vi "运维调试_采配水V4-华南所.vi"() -> ()   [LabVIEW 2016, in "PLC.lvlib"]
uses:
  PLC.lvlib
  control/switch.ctl
  <vilib>/Plasmionique/MB Master/MB_Master/MB_Master.lvclass
  <vilib>/Utility/miscctls.llb/LVPointTypeDef.ctl
  <vilib>/Plasmionique/MB Master/MB_Master_Serial/MB_Master_Serial.lvclass
  C:/Program Files (x86)/National Instruments/LabVIEW 2016/vi.lib/Plasmionique/MB Master/MB_Master/MB_Master.lvclass
  <vilib>/Plasmionique/MB Master/MB_Master_TCP/MB_Master_TCP.lvclass
  <vilib>/Instr/_visa.llb/VISA Configure Serial Port (Instr).vi
  <vilib>/Plasmionique/MB Master/MB Master.lvlib
panel:
  out "R138":i16 caption="水槽搅拌时间"
  out "R137":i16 caption="水槽润洗时间"
  out "X13":bool caption="三通道水槽3液位"
  out "X12":bool caption="三通道水槽2液位"
  out "X11":bool caption="三通道水槽1液位"
  in  "Y28":T1
  out "R41":i16
  in  "Y15":T1
  in  "Y16":T1
  in  "Y2":T1
  in  "Y3":T1
  in  "Y4":T1
  in  "Y5":T1
  in  "Y6":T1
  in  "Y7":T1
  in  "Y8":T1
  in  "Y9":T1
  in  "Y10":T1
  in  "Y11":T1
  in  "Y12":T1
  in  "Y0":T1
  in  "Y1":T1
  in  "Y13":T1
  in  "Y14":T1
  in  "Y17":T1
  in  "Y18":T1
  out "R13":u16
  out "R14":u16
  out "R15":u16
  out "R16":u16
  out "R17":u16
  out "R18":u16
  out "R19":u16
  out "R20":u16
  out "R21":u16
  out "R22":u16
  out "R23":u16
  out "R24":u16
  out "R25":u16
  out "R26":u16
  out "R27":u16
  out "R28":u16
  out "R29":u16
  out "R30":u16
  out "R31":u16
  in  "Y29":T1
  out "R42":i16
  in  "Y30":T1
  out "R43":u16
  in  "Y31":T1
  out "R44":u16
  in  "Y21":T1
  out "R34":u16
  in  "连接设置":bool
  in  "R136":u16(ring) caption="河水反冲洗模式" items=["泵保持", "泵交替"]
  out "R135":i16 caption="除藻时间"
  in  "R134":u16(ring) caption="除藻工作模式" items=["手动", "自动"]
  in  "R110":u16(ring) caption="反冲洗水体" items=["自来水", "河水"]
  in  "63μm反冲洗阀":bool
  out "供水压力":dbl format="%.4f"
  out "R111":i16 caption="三级水样池润洗时间"
  in  "三级过滤系统":bool
  out "R104":i16 caption="三级润洗时间"
  out "R103":i16 caption="二级润洗时间"
  out "R107":i16 caption="进气时间"
  out "Registers":u16[](array[numeric])
  out "R124":i16 caption="加标回收配水时间"
  in  "更新程序":T1
  out "R122":i16 caption="二级自来水清洗时间"
  out "R121":i16 caption="一级自来水清洗时间"
  out "R120":i16 caption="过滤自来水清洗时间"
  out "清洗次数":u16
  out "当前启动泵号":u16(ring) items=["1号泵", "2号泵"]
  out "R116":i16 caption="储水时间"
  in  "R113":u16(ring) caption="水箱储水水体" items=["自来水", "河水"]
  out "R112":i16 caption="二级水样池进样超时"
  out "配水压力":dbl format="%.4f"
  out "X2":bool caption="X1"
  out "采配水版本号":string
  out "R117":i16 caption="清洗频次设定"
  out "通讯故障":bool
  in  "R100":u16(ring) caption="采水泵工作模式" items=["泵1单泵单管路", "泵2单泵单管路", "潜水泵双泵双管路", "自吸泵双泵双管路"]
  out "X10":bool caption="氨氮水样池液位开关SL3"
  out "X9":bool caption="泵2过载报警_KM2"
  out "X8":bool caption="泵1过载报警_KM1"
  out "X7":bool caption="断电检测_PA"
  out "X6":bool caption="门禁开关_AS"
  out "X5":bool caption="烟雾检测_SA"
  out "X4":bool caption="浸水检测_WIA"
  out "X3":bool caption="水流开关_FS"
  out "X1":bool
  out "X0":bool caption="采样池液位开关_SL1"
  out "R109":i16 caption="外部反冲洗时间"
  out "R108":i16 caption="进样超时时间"
  out "R106":i16 caption="排液时间"
  out "R105":i16 caption="常规模式配水时间"
  out "R102":i16 caption="沉淀时间"
  out "R101":i16 caption="一级润洗时间"
  out "R2":i16
  out "R1":i16
  out "多列列表框":i32(listbox)
  in  "返回":T1
  in  "参数设置":T1
  in  "单步启动":T1
  in  "启动":T1
  in  "停止":T1
  out "集成报警信息":string
  # "s"
  # "流程计时："
  # "s"
  # "单步计时："
  # "MPa"
  # "配水压力："
  # "MPa"
  # "供水压力："
  # "S"
  # "S"
  # "S"
  # "S"
  # "S"
  # "S"
  # "S"
  # "S"
  # "S"
  # "S"
  # "S"
  # "S"
  # "S"
  # "次"
  # "S"
  # "S"
  # "S"
  # "S"
  # "S"
  # "S"
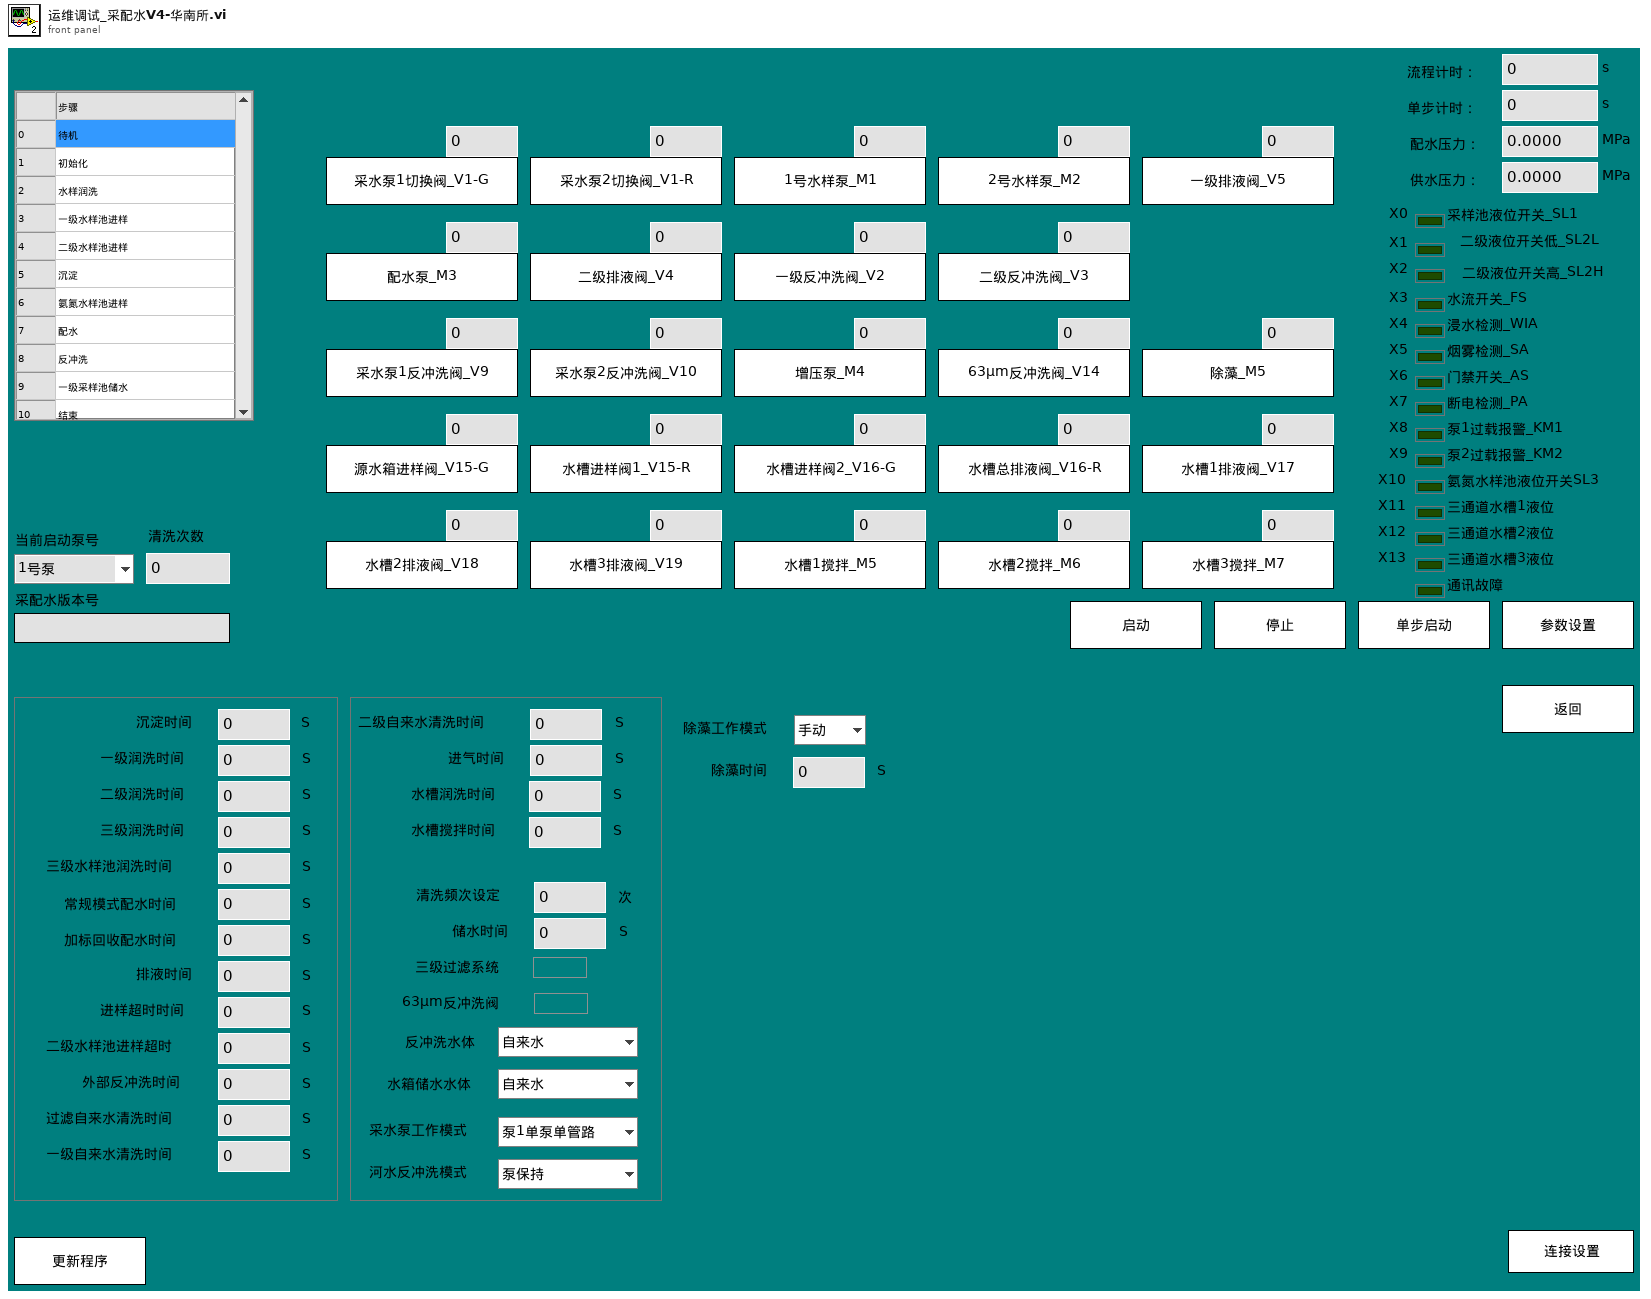
[diagram p1: front panel]
types:
  T1 = typedef "PLC.lvlib/switch.ctl" = bool
  T2 = typedef "参数.ctl" = cluster{"测试模式":enum16{"水样测试", "平行样测试", "集成干预测试", "加标回收"}, "参数启用":T3}
  T3 = typedef "启动参数.ctl" = cluster{"氨氮":bool, "总磷":bool, "总氮":bool, "多参数":bool, "CODmn":bool, "CODCr":bool, "氟化物":bool, "超标留样":bool, "重金属":bool, "挥发酚":bool}
  T4 = typedef "LVPointTypeDef.ctl" = cluster{"Horizontal":i16, "Vertical":i16}
  T5 = cluster{"命令":string, "数据":cluster{"starting address":u16, "holding register value":u16}}
  T6 = cluster{"R0":i16, "R1":i16, "R2":i16, "R3":i16, "R4":i16, "R5":i16, "R6":i16, "R7":i16, "R8":i16, "R9":i16, "R10":i16, "R11":i16, "R12":i16, "R13":i16, "R14":i16, "R15":i16, "R16":i16, "R17":i16, "R18":i16, "R19":i16, "R20":i16, "R21":i16, "R22":i16, "R23":i16, "R24":i16, "R25":i16, "R26":i16, "R27":i16, "R28":i16, "R29":i16, "R30":i16, "R31":i16, "R32":i16, "R33":i16, "R34":i16, "R35":i16, "R36":i16, "R37":i16, "R38":i16, "R39":i16, "R40":i16, "R41":i16, "R42":i16, "R43":i16, "R44":i16, "R45":i16, "R46":i16, "R47":i16, "R48":i16, "R49":i16, "R50":i16, "R51":i16, "R52":i16, "R53":i16, "R54":i16, "R55":i16, "R56":i16, "R57":i16, "R58":i16, "R59":i16, "R60":i16, "R61":i16, "R62":i16, "R63":i16, "R64":i16, "R65":i16, "R66":i16, "R67":i16, "R68":i16, "R69":i16, "R70":i16, "R71":i16, "R72":i16, "R73":i16, "R74":i16, "R75":i16, "R76":i16, "R77":i16, "R78":i16, "R79":i16}
  T7 = cluster{"seconds since 1Jan1904":timestamp, "table输入":string, string, "table输入":string}
  T8 = cluster{"命令":string, cluster{"starting address":u16, "holding register value":u16}}
  T9 = cluster{"命令":string, "数据":cluster{"starting address":u16, "holding register values":u16[]}}
  T10 = cluster{"命令":string, "data":cluster{"starting address":u16, "coil values":bool[]}}
  T11 = cluster{"测试模式":enum16{"水样测试", "平行样测试", "集成干预测试", "加标回收"}, "参数启用":T3}
  T12 = cluster{"baud rate (bps)":u32, "stop bits":u16, "parity":u16, "flow control":u16, "timeout":u32, "retries":i32}
  T13 = cluster{"starting address":u16, "holding register values":u16[]}
  T14 = cluster{"starting address":u16, "holding register value":u16}
  T15 = cluster{"starting address":u16, "coil values":bool[]}
  T16 = cluster{"连接类型":enum16{"串口", "TCP"}, "串口":string, "IP":string, "PORT":u16}
  T17 = cluster{"Registers[0]":u16, "Registers[1]":u16, "Registers[2]":u16, "Registers[3]":u16, "Registers[4]":u16, "Registers[5]":u16, "Registers[6]":u16, "Registers[7]":u16, "Registers[8]":u16, "Registers[9]":u16, "Registers[10]":u16, "Registers[11]":u16, "Registers[12]":u16, "Registers[13]":u16, "Registers[14]":u16, "Registers[15]":u16, "Registers[16]":u16, "Registers[17]":u16, "Registers[18]":u16, "Registers[19]":u16, "Registers[20]":u16, "Registers[21]":u16, "Registers[22]":u16, "Registers[23]":u16, "Registers[24]":u16, "Registers[25]":u16, "Registers[26]":u16, "Registers[27]":u16, "Registers[28]":u16, "Registers[29]":u16, "Registers[30]":u16, "Registers[31]":u16, "Registers[32]":u16, "Registers[33]":u16, "Registers[34]":u16, "Registers[35]":u16, "Registers[36]":u16, "Registers[37]":u16, "Registers[38]":u16, "Registers[39]":u16, "Registers[40]":u16, "Registers[41]":u16, "Registers[42]":u16, "Registers[43]":u16, "Registers[44]":u16, "Registers[45]":u16, "Registers[46]":u16, "Registers[47]":u16, "Registers[48]":u16, "Registers[49]":u16, "Registers[50]":u16, "Registers[51]":u16, "Registers[52]":u16, "Registers[53]":u16, "Registers[54]":u16, "Registers[55]":u16, "Registers[56]":u16, "Registers[57]":u16, "Registers[58]":u16, "Registers[59]":u16, "Registers[60]":u16, "Registers[61]":u16, "Registers[62]":u16, "Registers[63]":u16, "Registers[64]":u16, "Registers[65]":u16, "Registers[66]":u16, "Registers[67]":u16, "Registers[68]":u16, "Registers[69]":u16, "Registers[70]":u16, "Registers[71]":u16, "Registers[72]":u16, "Registers[73]":u16, "Registers[74]":u16, "Registers[75]":u16, "Registers[76]":u16, "Registers[77]":u16, "Registers[78]":u16, "Registers[79]":u16}
  T18 = cluster{"Registers[0]":u16, "Registers[1]":u16, "Registers[2]":u16, "Registers[3]":u16, "Registers[4]":u16, "Registers[5]":u16}
  T19 = cluster{"Registers[0]":u16, "Registers[1]":u16, "Registers[2]":u16, "Registers[3]":u16, "Registers[4]":u16, "Registers[5]":u16, "Registers[6]":u16, "Registers[7]":u16, "Registers[8]":u16, "Registers[9]":u16, "Registers[10]":u16, "Registers[11]":u16, "Registers[12]":u16, "Registers[13]":u16, "Registers[14]":u16, "Registers[15]":u16, "Registers[16]":u16, "Registers[17]":u16, "Registers[18]":u16, "Registers[19]":u16, "Registers[20]":u16, "Registers[21]":u16, "Registers[22]":u16, "Registers[23]":u16, "Registers[24]":u16, "Registers[25]":u16, "Registers[26]":u16, "Registers[27]":u16, "Registers[28]":u16, "Registers[29]":u16, "Registers[30]":u16, "Registers[31]":u16, "Registers[32]":u16, "Registers[33]":u16, "Registers[34]":u16, "Registers[35]":u16, "Registers[36]":u16}
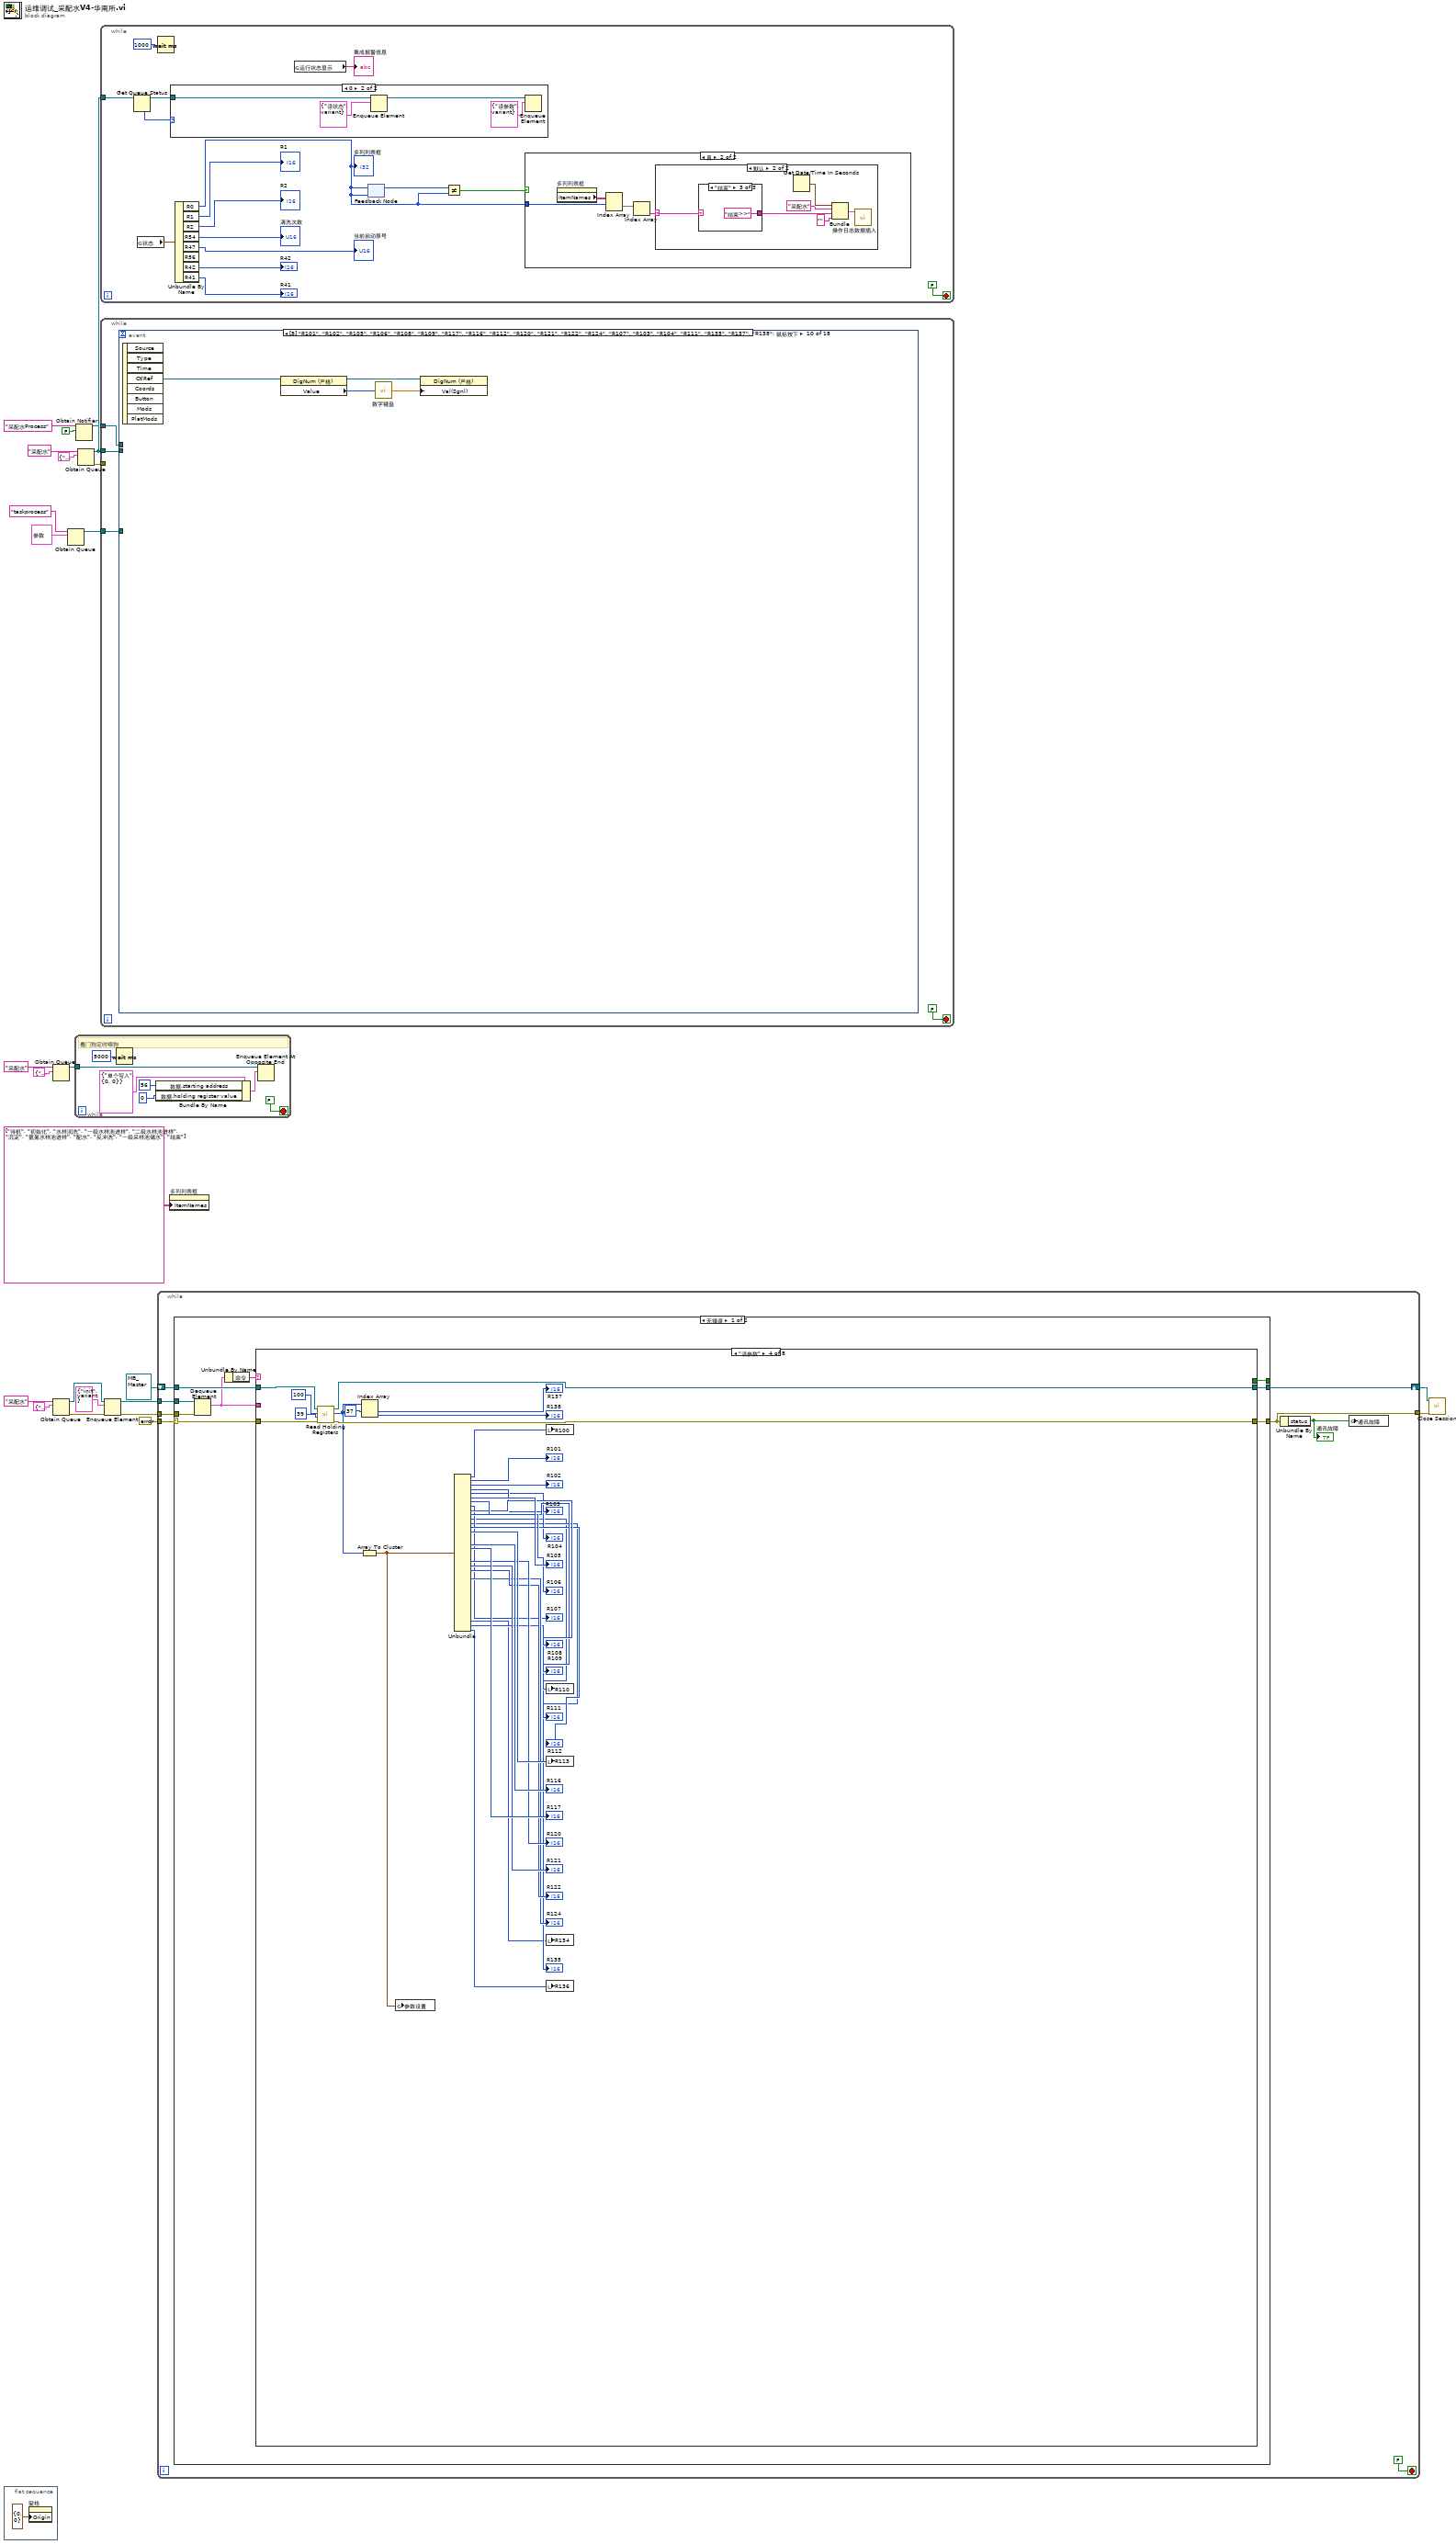
[diagram p0: block diagram]
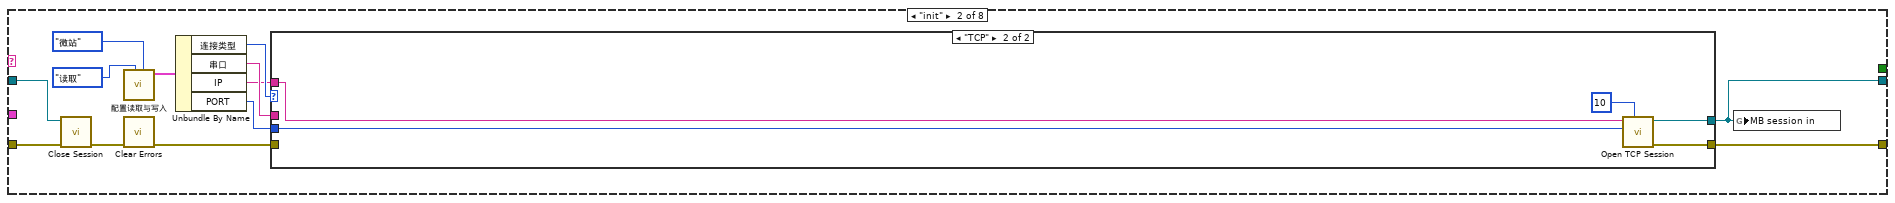
[diagram p3: hidden frame]
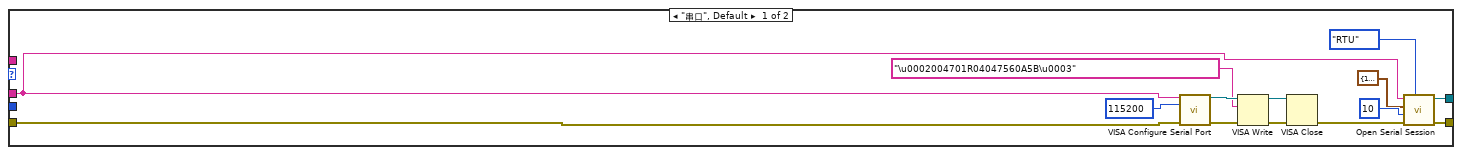
[diagram p4: hidden frame]
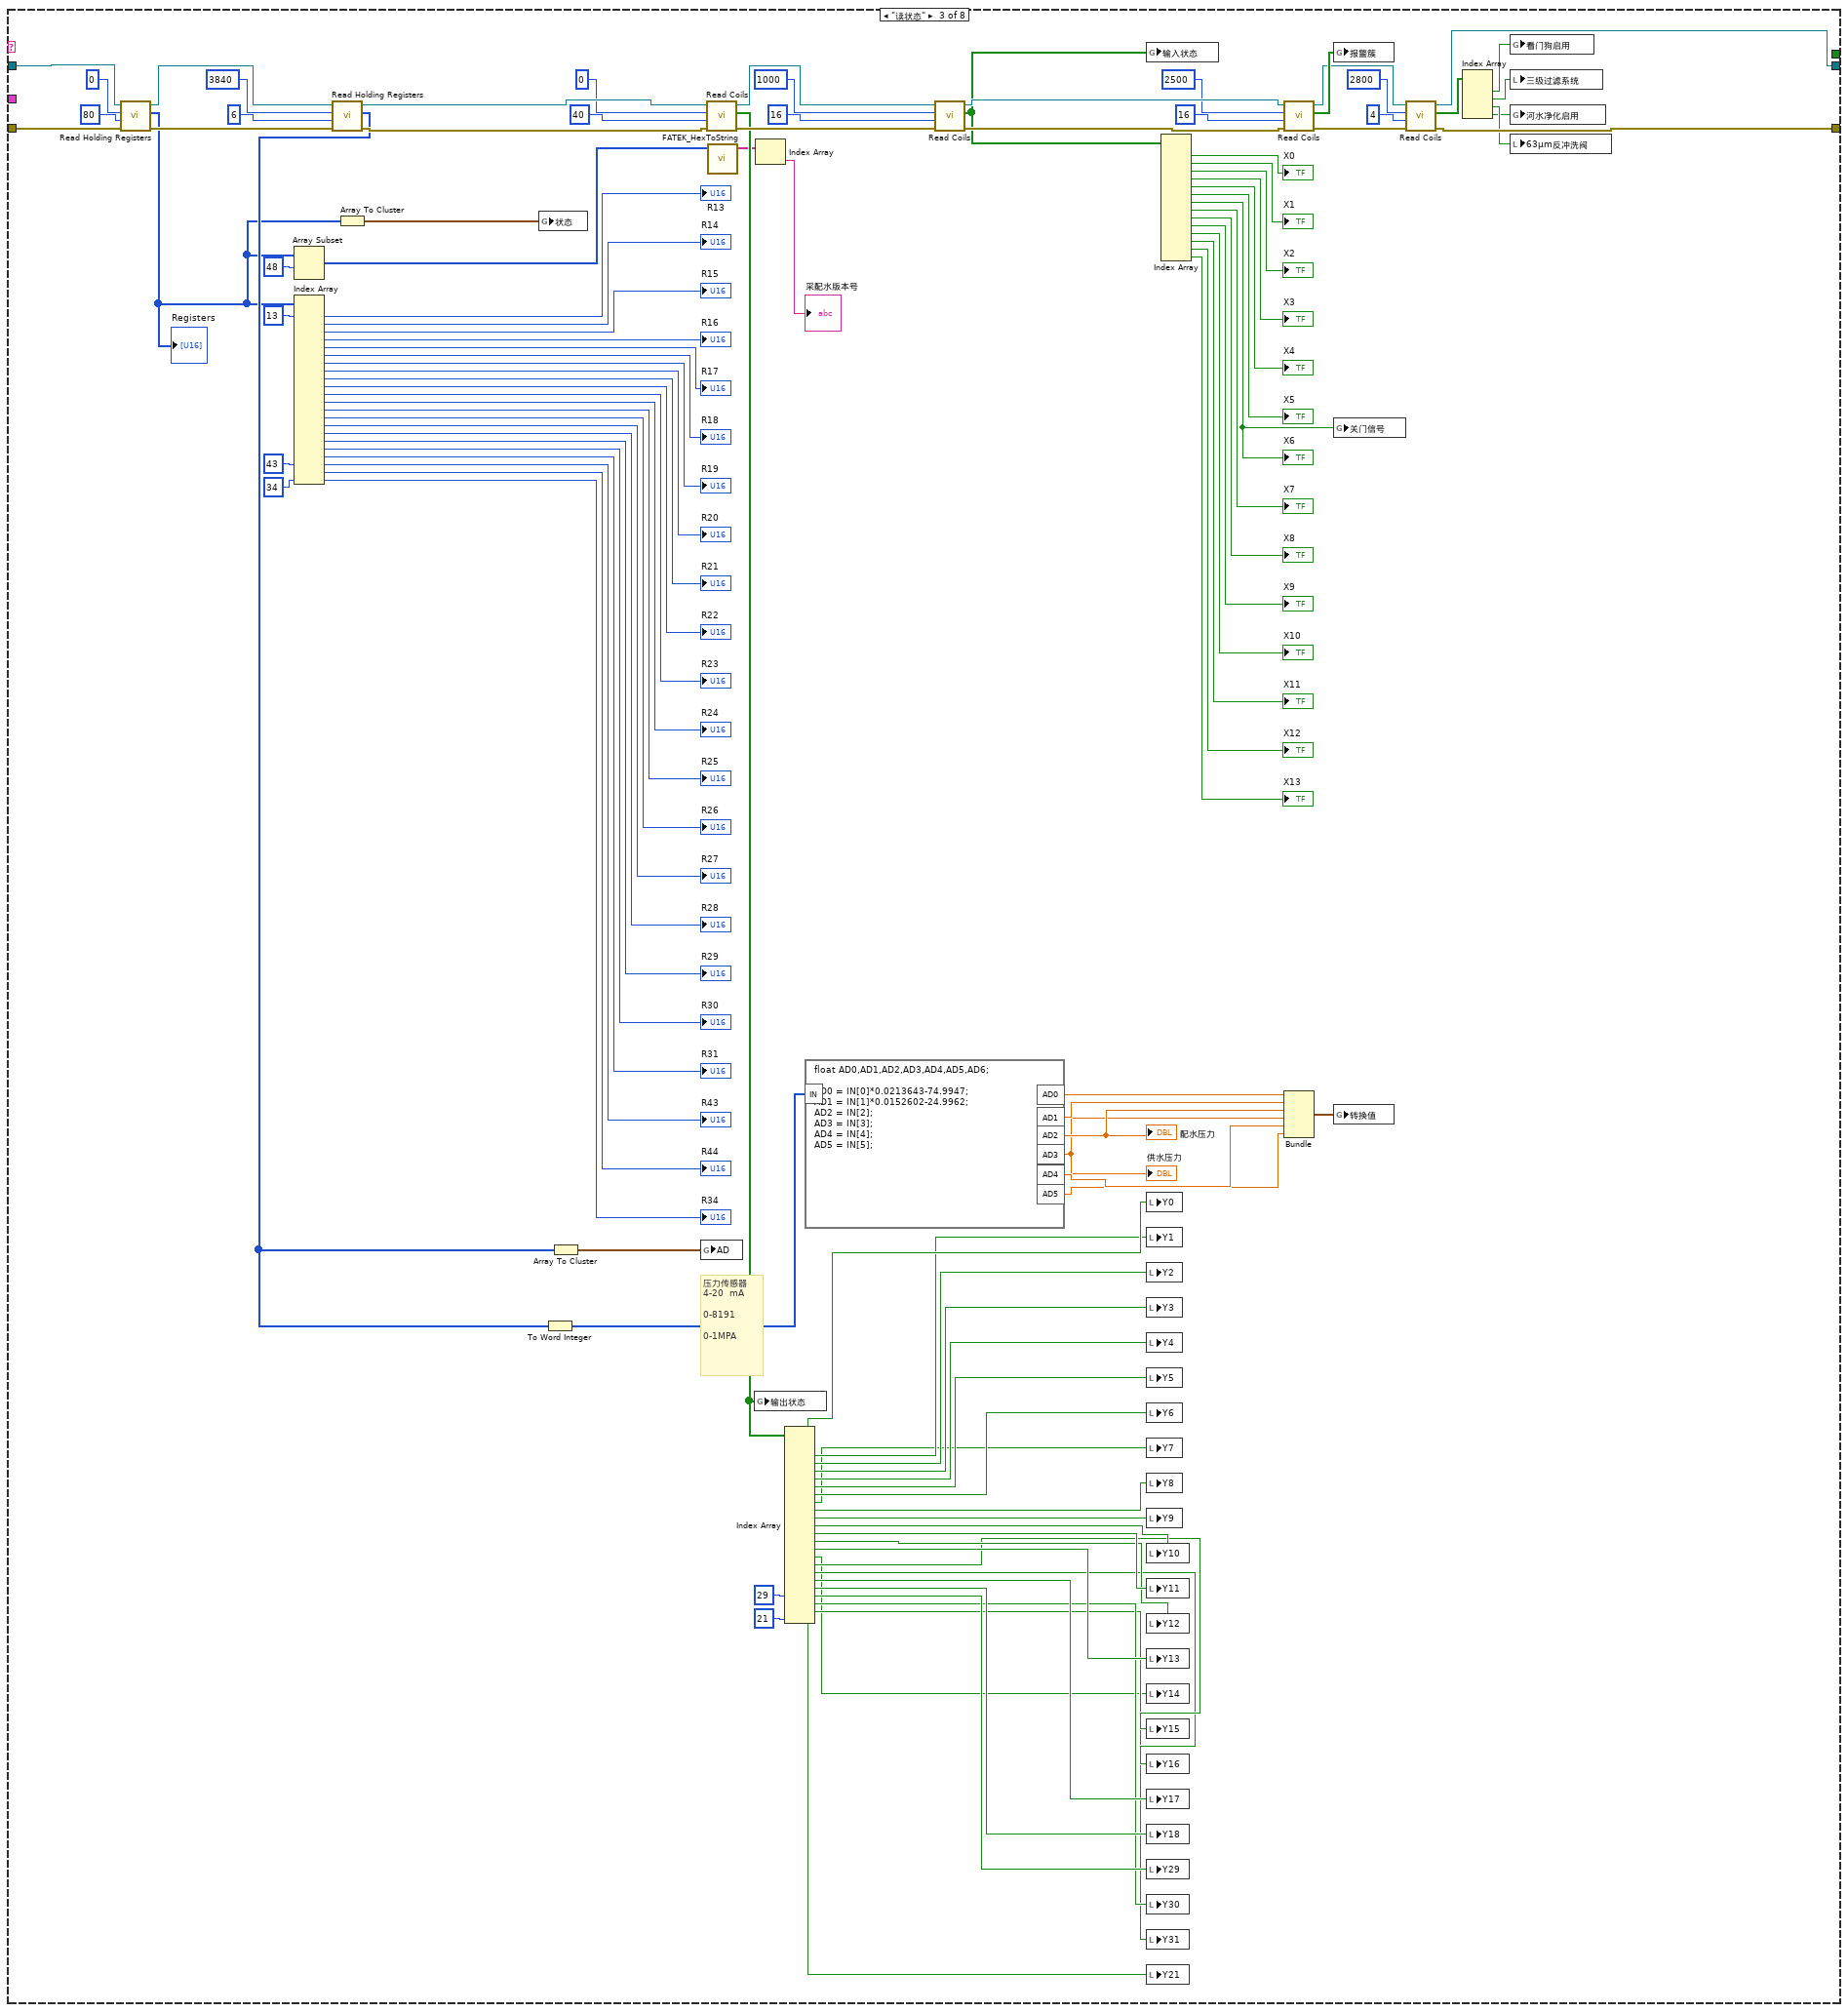
[diagram p5: hidden frame]
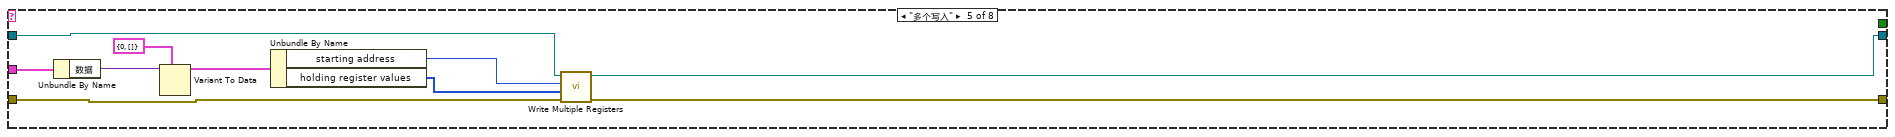
[diagram p6: hidden frame]
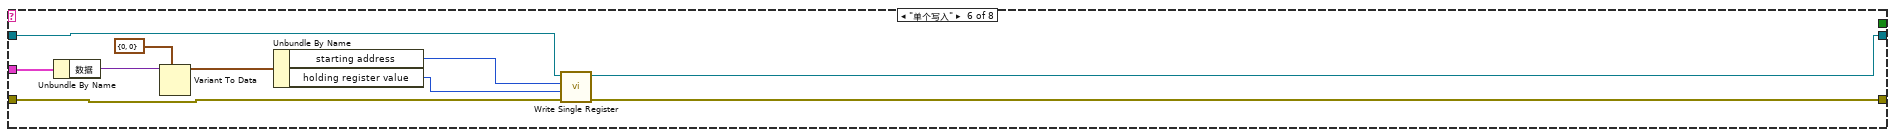
[diagram p7: hidden frame]
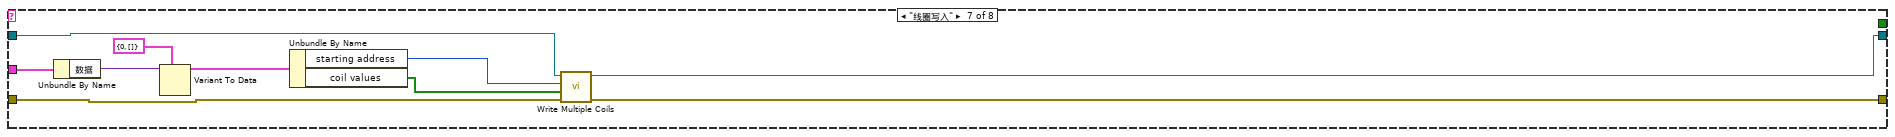
[diagram p8: hidden frame]
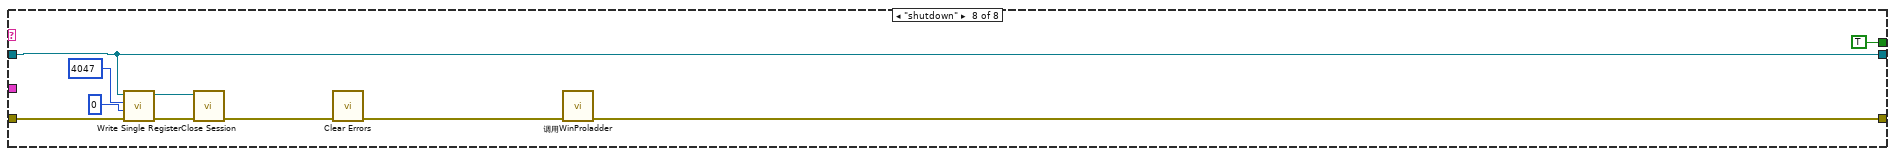
[diagram p9: hidden frame]
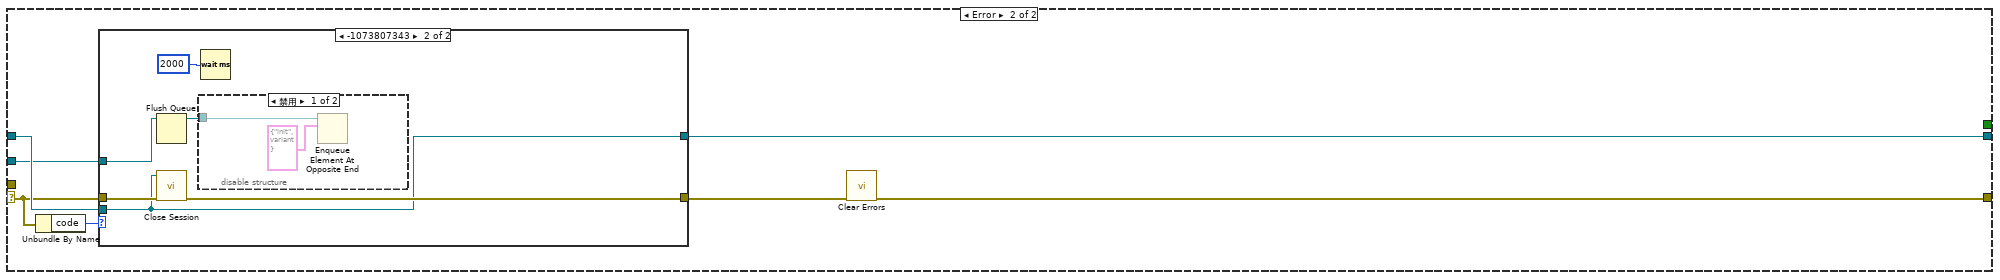
[diagram p10: hidden frame]
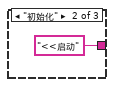
[diagram p17: hidden frame]
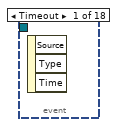
[diagram p18: hidden frame]
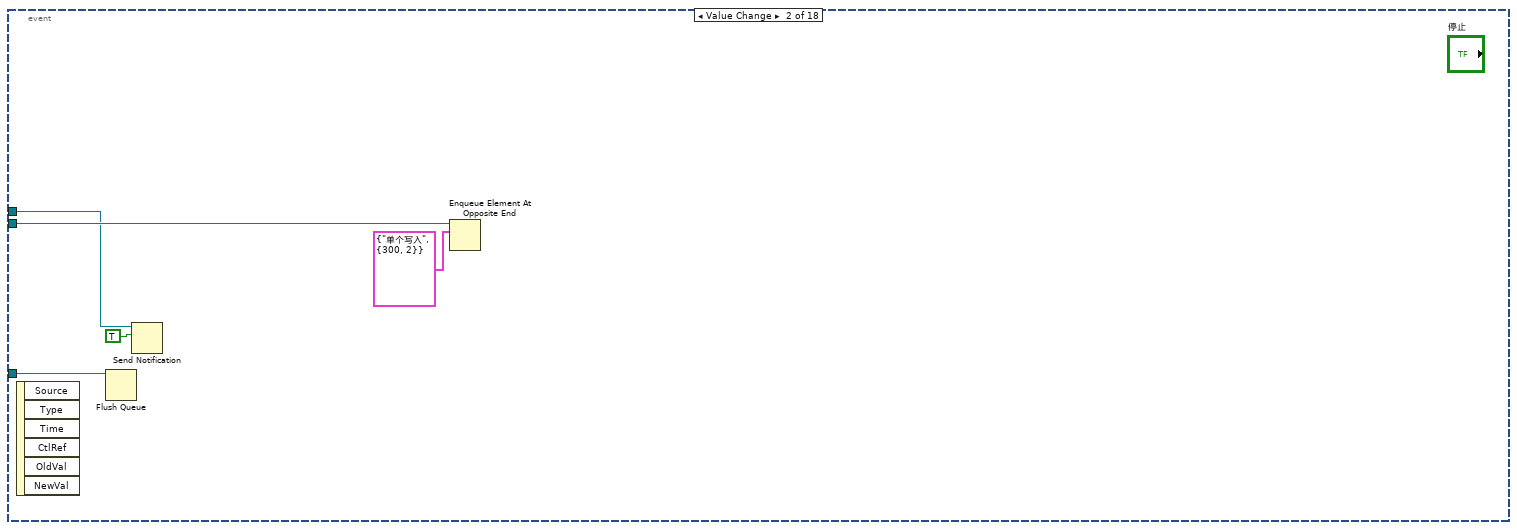
[diagram p19: hidden frame]
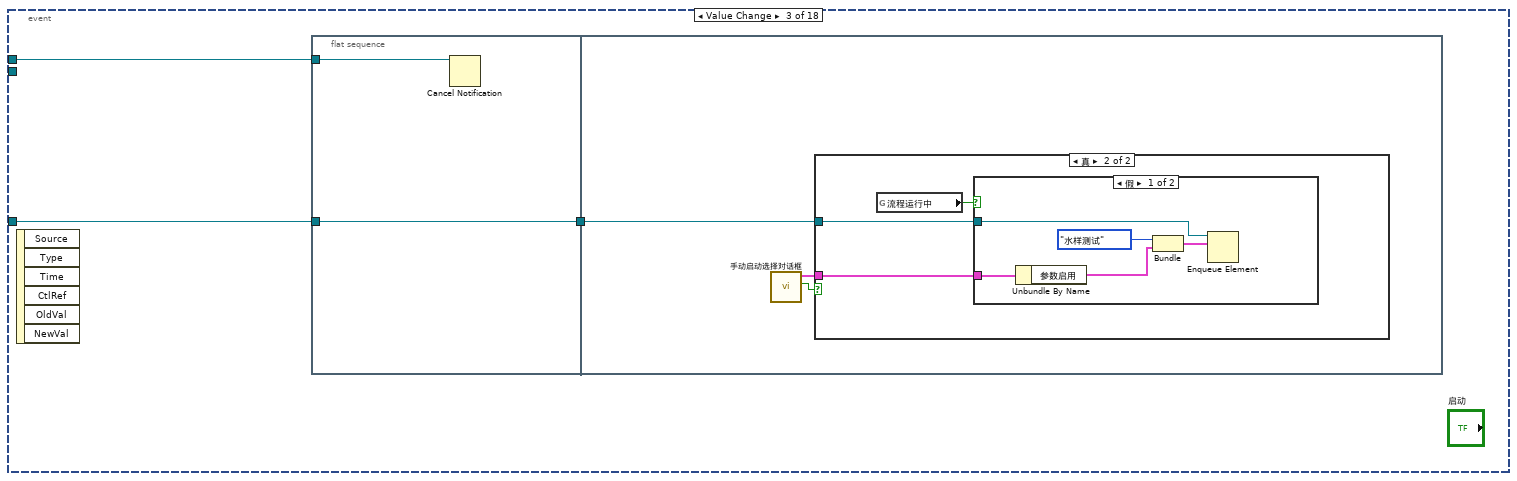
[diagram p20: hidden frame]
diagram:
  n1 = flat-sequence {
    frame #0 {
      n2 = property on="窗格" class="Pane"("Origin"=T4 {"Horizontal"=0, "Vertical"=0} ("原点")) -> ()  [unwired: 2 in, 2 out]
    }
  }
  n3 = Obtain Queue(name (unnamed)="采配水" ("名称（未命名）"), element data type=cluster{"命令":string, "数据":variant} {"命令"="", "数据"=variant}) -> (queue out=w4:refnum<queue>)  [unwired: 3 in, 2 out]
  n4 = Obtain Queue(name (unnamed)="采配水" ("名称（未命名）"), element data type=cluster{"命令":string, "数据":variant} {"命令"="", "数据"=variant}) -> (queue out=w15:refnum<queue>, error out=w14:errorcluster)  [unwired: 3 in, 1 out]
  n5 = Obtain Queue(name (unnamed)="taskprocess" ("名称（未命名）"), element data type=T2 {"测试模式"=enum."水样测试", "参数启用"={"氨氮"=FALSE, "总磷"=FALSE, "总氮"=FALSE, "多参数"=FALSE, "CODmn"=FALSE, "CODCr"=FALSE, "氟化物"=FALSE, "超标留样"=FALSE, "重金属"=FALSE, "挥发酚"=FALSE}} ("参数")) -> (queue out=w2:refnum<queue>)  [unwired: 3 in, 2 out]
  n6 = while {
    tunnel: w4 -> [w31]
    stop <- FALSE stop-if-true
    # "看门狗定时喂狗"
    n7 = Wait (ms)(milliseconds to wait=u32 5000 ("等待时间（毫秒）")) -> ()  [unwired: 1 out]
    n8 = Bundle By Name(cluster=T5 {"命令"="单个写入", "数据"={"starting address"=0, "holding register value"=0}} ("元素"), "数据.starting address"=u16 56, "数据.holding register value"=u16 0) -> (w32:T5)
    n9 = Enqueue Element At Opposite End(queue=w31, element=w32) -> ()  [unwired: 2 in, 3 out]
  }
  n10 = Obtain Notifier(name (unnamed)="采配水Process" ("名称（未命名）"), notification data type=FALSE) -> (notifier out=w18:refnum<notifier>)  [unwired: 2 in, 2 out]
  n11 = Obtain Queue(name (unnamed)="采配水" ("名称（未命名）"), element data type=cluster{"命令":string, "数据":variant} {"命令"="", "数据"=variant}) -> (queue out=w22:refnum<queue>, error out=w23:errorcluster)  [unwired: 3 in, 1 out]
  n12 = while {
    tunnel: w22 -> [w48]
    stop <- FALSE stop-if-true
    n13 = Get Queue Status(queue=w48) -> (queue out=w36:refnum<queue>, # elements in queue=w35:i32)  [unwired: 2 in, 6 out]
    n14 = global read "采配水全局变量.vi" "状态"() -> (w47:T6)
    n15 = Wait (ms)(milliseconds to wait=u32 1000 ("等待时间（毫秒）")) -> ()  [unwired: 1 out]
    n16 = case shown="0" w35 {
      tunnel: w36 -> [_ w53]
      frame Default {
      }
      frame 0 {
        n17 = Enqueue Element(queue=w53, element=cluster{"命令":string, "数据":variant} {"命令"="读状态", "数据"=variant} ("元素")) -> (queue out=w50:refnum<queue>)  [unwired: 2 in, 2 out]
        n18 = Enqueue Element(queue=w50, element=cluster{"命令":string, "数据":variant} {"命令"="读参数", "数据"=variant} ("元素")) -> ()  [unwired: 2 in, 3 out]
      }
    }
    n19 = Unbundle By Name(w47) -> ("R0"=w40:i16, "R1"=→"R1":i16, "R2"=→"R2":i16, "R54"=→"清洗次数":i16, "R47"=→"当前启动泵号":i16, "R42"=→"R42":i16, "R41"=→"R41":i16)  [unwired: 1 out]
    "多列列表框" <- w40
    n20 = global read "采配水全局变量.vi" "运行状态显示"() -> (→"集成报警信息":string)
    n21 = feedback-in #1(w40) -> ()
    n22 = feedback #1(w40) -> (w41:i16)
    n23 = Not Equal?(x=w41, y=w40) -> (x != y?=w44:bool)
    n24 = case shown="真" w44 {
      tunnel: w40 -> [_ w56]
      frame False {
      }
      frame True {
        n25 = property on="多列列表框" class="MCListbox (严格)"() -> ("ItemNames"=w57:string[][])  [unwired: 2 in, 2 out]
        n26 = Index Array(array=w57, index (row)=w56) -> (element=w55:string[])  [unwired: 1 in]
        n27 = Index Array(array=w55) -> (element=w54:string)  [unwired: 1 in]
        n28 = case shown="默认" w54 {
          selector: w54 -> [_ w60]
          frame "待机" {
          }
          frame Default {
            n29 = case shown="\"结束\"" w60 {
              selector: w60 -> [w64 _ _]
              tunnel: [w64 "<<启动" "结束>>"] -> w59
              frame Default {
              }
              frame "初始化" {
              }
              frame "结束" {
              }
            }
            n30 = Get Date/Time In Seconds() -> (seconds since 1Jan1904=w63:timestamp)
            n31 = Bundle("seconds since 1Jan1904"=w63, "table输入"="采配水", w59, "table输入"="") -> (w58:T7)  [unwired: 1 in]
            n32 = call "操作日志数据插入.vi"("data"=w58) -> ()  [unwired: 9 in, 1 out]
          }
        }
      }
    }
  }
  n33 = while {
    tunnel: w22 -> [w69]
    tunnel: w23 -> [_]
    tunnel: w18 -> [w68]
    tunnel: w2 -> [w67]
    stop <- FALSE stop-if-true
    n34 = event shown="[9] \"R101\", \"R102\", \"R105\", \"R106\", \"R108\", \"R109\", \"R117\", \"R116\", \"R112\", \"R120\", \"R121\", \"R122\", \"R124\", \"R107\", \"R103\", \"R104\", \"R111\", \"R135\", \"R137\", \"R138\": 鼠标按下" {
      selector: _ -> [_ _ _ _ _ _ _ _ _ _ _ _ _ _ _ _ _ _]
      dyn-events: _ -> [_ _ _ _ _ _ _ _ _ _ _ _ _ _ _ _ _ _]
      timeout: _ -> [_ _ _ _ _ _ _ _ _ _ _ _ _ _ _ _ _ _]
      tunnel: w69 -> [_ w74 _ w96 w115 w124 w129 w139 w144 _ _ _ w177 w180 w188 w193 w198 w204]
      tunnel: w68 -> [_ w73 w78 _ _ _ _ _ _ _ _ _ _ _ _ _ _ _]
      tunnel: w67 -> [_ w71 w76 _ _ _ _ _ _ _ _ _ _ _ _ _ _ _]
      event Timeout {
        n35 = event-data() -> ()  [unwired: 1 in, 3 out]
      }
      event Value Change {
        n36 = event-data() -> ()  [unwired: 1 in, 6 out]
        n37 = Flush Queue(queue=w71) -> ()  [unwired: 1 in, 3 out]
        n38 = Send Notification(notification=TRUE ("通知"), notifier=w73) -> ()  [unwired: 1 in, 2 out]
        n39 = Enqueue Element At Opposite End(queue=w74, element=T8 {"命令"="单个写入", {"starting address"=300, "holding register value"=2}} ("元素")) -> ()  [unwired: 2 in, 3 out]
      }
      event Value Change {
        n40 = event-data() -> ()  [unwired: 1 in, 6 out]
        n41 = flat-sequence {
          tunnel: w78 -> [w80]
          tunnel: [w79] -> w77
          tunnel: w76 -> [w79]
          tunnel: w77 -> [w81]
          frame #0 {
            n42 = Cancel Notification(0:w80) -> ()  [unwired: 1 in, 3 out]
          }
          frame #1 {
            n43 = call "手动启动选择对话框.vi"() -> ("确定"=w83:bool, "输出簇"=w82:cluster{"参数启用":T3})  [unwired: 10 in]
            n44 = case shown="真" w83 {
              tunnel: w82 -> [_ w86]
              tunnel: w81 -> [_ w85]
              frame False {
              }
              frame True {
                n45 = global read "采配水全局变量.vi" "流程运行中"() -> (w84:bool)
                n46 = case shown="假" w84 {
                  tunnel: w86 -> [w89 _]
                  tunnel: w85 -> [w91 _]
                  frame False {
                    n47 = Unbundle By Name(w89) -> ("参数启用"=w88:T3)
                    n48 = Bundle("测试模式"=enum16{"水样测试", "平行样测试", "集成干预测试", "加标回收"}."水样测试", "参数启用"=w88) -> (w87:T11)  [unwired: 1 in]
                    n49 = Enqueue Element(queue=w91, element=w87) -> ()  [unwired: 2 in, 3 out]
                  }
                  frame True {
                    n50 = One Button Dialog(message="流程已启动，无需重复启动！" ("消息")) -> ()  [unwired: 1 in, 1 out]
                  }
                }
              }
            }
          }
        }
      }
      event Value Change {
        n51 = event-data() -> ()  [unwired: 1 in, 6 out]
        n52 = call "单步启动对话框.vi"() -> ("单步启动步骤输出"=w93:u16)  [unwired: 11 in]
        n53 = Bundle By Name(cluster=T5 {"命令"="单个写入", "数据"={"starting address"=301, "holding register value"=0}} ("元素"), "数据.holding register value"=w93) -> (w94:T5)
        n54 = Enqueue Element At Opposite End(queue=w96, element=w94) -> ()  [unwired: 2 in, 3 out]
      }
      event "R101", "R102", "R105", "R106", "R108", "R109", "R100", "R112", "R113", "R103", "R104", "R107", "R111", "R110": Value Change {
        n55 = event-data() -> ()  [unwired: 1 in, 6 out]
        n56 = local read "R101"() -> (w111:i16)
        n57 = local read "R102"() -> (w110:i16)
        n58 = local read "R103"() -> (w100:i16)
        n59 = local read "R104"() -> (w99:i16)
        n60 = local read "R105"() -> (w109:i16)
        n61 = local read "R106"() -> (w108:i16)
        n62 = local read "R107"() -> (w107:i16)
        n63 = local read "R108"() -> (w106:i16)
        n64 = local read "R109"() -> (w104:i16)
        n65 = local read "R111"() -> (w98:i16)
        n66 = local read "R112"() -> (w102:i16)
        n67 = Build Array("R100", w111, w110, w100, w99, w109, w108, w107, w106, w104, "R110", w98, w102, "R113") -> (w103:u16[])
        n68 = Bundle By Name(cluster=T9 {"命令"="多个写入", "数据"={"starting address"=0, "holding register values"=[]}} ("元素"), "数据.starting address"=u16 100, "数据.holding register values"=w103) -> (w112:T9)
        n69 = Enqueue Element At Opposite End(queue=w115, element=w112) -> ()  [unwired: 2 in, 3 out]
      }
      event "R116", "R117", "R120", "R121", "R122": Value Change {
        n70 = event-data() -> ()  [unwired: 1 in, 6 out]
        n71 = local read "R116"() -> (w122:i16)
        n72 = local read "R117"() -> (w121:i16)
        n73 = local read "R120"() -> (w120:i16)
        n74 = local read "R121"() -> (w119:i16)
        n75 = local read "R122"() -> (w118:i16)
        n76 = Build Array(w122, w121, i16 0 ("元素"), i16 0 ("R116"), w120, w119, w118) -> (w123:i16[])
        n77 = Bundle By Name(cluster=T9 {"命令"="多个写入", "数据"={"starting address"=0, "holding register values"=[]}} ("元素"), "数据.starting address"=u16 116, "数据.holding register values"=w123) -> (w125:T9)
        n78 = Enqueue Element At Opposite End(queue=w124, element=w125) -> ()  [unwired: 2 in, 3 out]
      }
      event "R124": Value Change {
        n79 = event-data() -> ("NewVal"=w128:i16)  [unwired: 1 in, 5 out]
        n80 = Build Array(w128) -> (w130:i16[])
        n81 = Bundle By Name(cluster=T9 {"命令"="多个写入", "数据"={"starting address"=0, "holding register values"=[]}} ("元素"), "数据.starting address"=u16 124, "数据.holding register values"=w130) -> (w131:T9)
        n82 = Enqueue Element At Opposite End(queue=w129, element=w131) -> ()  [unwired: 2 in, 3 out]
      }
      event "R134", "R135", "R136", "R137", "R138": Value Change {
        n83 = event-data() -> ()  [unwired: 1 in, 6 out]
        n84 = local read "R135"() -> (w137:i16)
        n85 = local read "R137"() -> (w135:i16)
        n86 = local read "R138"() -> (w134:i16)
        n87 = Build Array("R134", w137, "R136", w135, w134) -> (w140:u16[])
        n88 = Bundle By Name(cluster=T9 {"命令"="多个写入", "数据"={"starting address"=0, "holding register values"=[]}} ("元素"), "数据.starting address"=u16 134, "数据.holding register values"=w140) -> (w141:T9)
        n89 = Enqueue Element At Opposite End(queue=w139, element=w141) -> ()  [unwired: 2 in, 3 out]
      }
      event "连接设置": Value Change {
        n90 = event-data() -> ()  [unwired: 1 in, 6 out]
        n91 = call "连接配置对话框.vi"("类别"=enum16{"微站", "固定站"}."微站") -> ("check？"=w146:bool)  [unwired: 18 in]
        n92 = case shown="真" w146 {
          tunnel: w144 -> [_ w148]
          frame False {
          }
          frame True {
            n93 = Enqueue Element(queue=w148, element=cluster{"命令":string, "数据":variant} {"命令"="init", "数据"=variant} ("元素")) -> ()  [unwired: 2 in, 3 out]
          }
        }
      }
      event "R101", "R102", "R105", "R106", "R108", "R109", "R117", "R116", "R112", "R120", "R121", "R122", "R124", "R107", "R103", "R104", "R111", "R135", "R137", "R138": Mouse Down {
        n94 = event-data() -> ("CtlRef"=w152:refnum<vi>)  [unwired: 1 in, 7 out]
        n95 = property class="DigNum (严格)"(reference=w152) -> (reference out=w150:refnum<vi>, "Value"=w151:i16)  [unwired: 1 in, 1 out]
        n96 = call "数字键盘.vi"("OldNumber"=w151) -> ("NewNumber"=w149:sgl)
        n97 = property class="DigNum (严格)"(reference=w150, "Val(Sgnl)"=w149) -> ()  [unwired: 1 in, 2 out]
      }
      event Value Change {
        n98 = event-data() -> ()  [unwired: 1 in, 6 out]
        n99 = property on="窗格" class="Pane"("Origin"=T4 {"Horizontal"=0, "Vertical"=628} ("原点")) -> ()  [unwired: 2 in, 2 out]
      }
      event Value Change {
        n100 = event-data() -> ()  [unwired: 1 in, 6 out]
        n101 = property on="窗格" class="Pane"("Origin"=T4 {"Horizontal"=0, "Vertical"=0} ("原点")) -> ()  [unwired: 2 in, 2 out]
      }
      event Value Change {
        n102 = event-data() -> ()  [unwired: 1 in, 6 out]
        n103 = Build Array("Y0", "Y1", "Y2", "Y3", "Y4", "Y5", "Y6", "Y7", "Y8", "Y9", "Y10", "Y11", "Y12", "Y13", "Y14", "Y15", "Y16", "Y17", "Y18") -> (w170:T1[])
        n104 = Bundle By Name(cluster=T10 {"命令"="线圈写入", "data"={"starting address"=2400, "coil values"=[]}} ("元素"), "data.coil values"=w170) -> (w171:T10)
        n105 = Enqueue Element(queue=w177, element=w171) -> ()  [unwired: 2 in, 3 out]
      }
      event Value Change {
        n106 = event-data() -> ()  [unwired: 1 in, 6 out]
        n107 = Build Array("Y21") -> (w178:T1[])
        n108 = Bundle By Name(cluster=T10 {"命令"="线圈写入", "data"={"starting address"=2451, "coil values"=[]}} ("元素"), "data.coil values"=w178) -> (w181:T10)
        n109 = Enqueue Element(queue=w180, element=w181) -> ()  [unwired: 2 in, 3 out]
      }
      event Value Change {
        n110 = event-data() -> ()  [unwired: 1 in, 6 out]
        n111 = Build Array("Y28", "Y29", "Y30", "Y31") -> (w187:T1[])
        n112 = Bundle By Name(cluster=T10 {"命令"="线圈写入", "data"={"starting address"=2429, "coil values"=[]}} ("元素"), "data.coil values"=w187) -> (w189:T10)
        n113 = Enqueue Element(queue=w188, element=w189) -> ()  [unwired: 2 in, 3 out]
      }
      event "三级过滤系统": Value Change {
        n114 = event-data() -> ()  [unwired: 1 in, 6 out]
        n115 = Build Array("三级过滤系统") -> (w191:bool[])
        n116 = Bundle By Name(cluster=T10 {"命令"="线圈写入", "data"={"starting address"=2801, "coil values"=[]}} ("元素"), "data.coil values"=w191) -> (w194:T10)
        n117 = Enqueue Element(queue=w193, element=w194) -> ()  [unwired: 2 in, 3 out]
      }
      event "63μm反冲洗阀": Value Change {
        n118 = event-data() -> ()  [unwired: 1 in, 6 out]
        n119 = Build Array("63μm反冲洗阀") -> (w197:bool[])
        n120 = Bundle By Name(cluster=T10 {"命令"="线圈写入", "data"={"starting address"=2802, "coil values"=[]}} ("元素"), "data.coil values"=w197) -> (w199:T10)
        n121 = Enqueue Element(queue=w198, element=w199) -> ()  [unwired: 2 in, 3 out]
      }
      event Value Change {
        n122 = event-data() -> ("NewVal"=w201:T1)  [unwired: 1 in, 5 out]
        n123 = case shown="真" w201 {
          tunnel: [cluster{"命令":string, "数据":variant} {"命令"="init", "数据"=variant} ("元素") w208] -> w203
          frame False {
          }
          frame True {
            n124 = Two Button Dialog(message="警告，非专业人士请勿进行此操作！！！\n请确认是否释放串口？" ("消息")) -> (T button?=w207:bool)  [unwired: 2 in]
            n125 = case shown="真" w207 {
              tunnel: [_ cluster{"命令":string, "数据":variant} {"命令"="shutdown", "数据"=variant} ("元素")] -> w208
              frame False {
                n126 = local write "更新程序"(FALSE ("释放串口")) -> ()
              }
              frame True {
              }
            }
          }
        }
        n127 = Flush Queue(queue=w204) -> (queue out=w202:refnum<queue>)  [unwired: 1 in, 2 out]
        n128 = Enqueue Element(queue=w202, element=w203) -> ()  [unwired: 2 in, 3 out]
      }
    }
  }
  n129 = Enqueue Element(queue=w15, element=cluster{"命令":string, "数据":variant} {"命令"="init", "数据"=variant} ("元素"), error in (no error)=w14) -> (queue out=w10:refnum<queue>, error out=w12:errorcluster)  [unwired: 1 in, 1 out]
  n130 = while {
    tunnel: w10 -> [w215]
    tunnel: w12 -> [w214]
    shift-right: [w218] -> w7
    shift-left: refnum<class "MB_Master.lvclass"> refnum ("MB session in") -> [w217]
    tunnel: errorcluster {"status"=FALSE, "code"=0, "source"=""} ("error out") -> [w216]
    tunnel: [w213] -> w8
    stop <- FALSE stop-if-true
    n131 = case shown="无错误" w216 {
      selector: w216 -> [w224 w454]
      tunnel: [w227 w453] -> w218
      tunnel: w217 -> [w226 w455]
      tunnel: [w225 w451] -> w213
      tunnel: w215 -> [w221 w450]
      tunnel: w214 -> [w220 _]
      tunnel: [w222 _] -> _
      frame No Error {
        n132 = Dequeue Element(queue=w221, error in (no error)=w220) -> (element=w219:cluster{"命令":string, "数据":variant})  [unwired: 1 in, 3 out]
        n133 = Unbundle By Name(w219) -> ("命令"=w223:string)
        n134 = case shown="\"读参数\"" w223 {
          tunnel: [w229 w232 w307 w405 w416 w426 w436 w447] -> w227
          tunnel: w226 -> [w229 w240 w366 w409 w419 w429 w439 w447]
          tunnel: [w228 w231 w298 w404 w417 w427 w437 w440] -> w225
          tunnel: w224 -> [w228 w242 w369 w408 w418 w428 w438 w443]
          tunnel: [_ _ _ _ _ _ _ TRUE] -> w222
          tunnel: w219 -> [_ _ _ _ w415 w425 w435 _]
          frame "idle", Default {
          }
          frame "init" {
            n135 = call-dynamic "Close Session.vi"("error in (no error)"=w242, "MB session in"=w240) -> ("error out"=w241:errorcluster)  [unwired: 9 in]
            n136 = call "配置读取与写入.vi"("类别"=enum16{"微站", "固定站"}."微站", "功能"=enum16{"读取", "写入"}."读取") -> ("连接配置 2"=w238:T16)  [unwired: 8 in, 1 out]
            n137 = call <vilib>:"Clear Errors.vi"("error in (no error)"=w241) -> ("error out"=w230:errorcluster)  [unwired: 5 in, 1 out]
            n138 = Unbundle By Name(w238) -> ("连接类型"=w235:enum16{"串口", "TCP"}, "串口"=w237:string, "IP"=w234:string, "PORT"=w233:u16)
            n139 = case shown="\"TCP\"" w235 {
              tunnel: [w256 w258] -> w231
              tunnel: w230 -> [w246 _]
              tunnel: [w244 w259] -> w232
              tunnel: w237 -> [w243 _]
              tunnel: w234 -> [_ w261]
              tunnel: w233 -> [_ w260]
              frame "串口", Default {
                n140 = call-poly "VISA Configure Serial Port"("VISA resource name"=w243, "baud rate (9600)"=u32 115200, "error in (no error)"=w246) -> ("VISA resource name out"=w252:refnum<visa-resource-name>, "error out"=w251:errorcluster)  [unwired: 11 in]
                n141 = VISA Write(VISA resource name=w252, write buffer="\u0002004701R04047560A5B\u0003" ("写入缓冲区"), error in (no error)=w251) -> (VISA resource name out=w250:refnum<visa-resource-name>, error out=w249:errorcluster)  [unwired: 1 out]
                n142 = VISA Close(VISA resource name=w250, error in (no error)=w249) -> (error out=w245:errorcluster)
                n143 = call <vilib>:"Open Serial Session.vi"("Mode (RTU)"=enum16{"RTU", "ASCII"}."RTU", "Error in"=w245, "Slave ID"=u8 10, "Serial Config"=T12 {"baud rate (bps)"=115200, "stop bits"=10, "parity"=0, "flow control"=0, "timeout"=500, "retries"=1}, "VISA Resource"=w243) -> ("Error out"=w256:errorcluster, "MB_Serial session"=w244:refnum<class "MB_Master_Serial.lvclass">)  [unwired: 5 in]
              }
              frame "TCP" {
                n144 = call <vilib>:"Open TCP Session.vi"("Slave ID (255)"=u8 10, "Port (502)"=w260, "IP Address"=w261) -> ("error out"=w258:errorcluster, "MB_TCP session"=w259:refnum<class "MB_Master_TCP.lvclass">)  [unwired: 7 in]
              }
            }
            n145 = global write "采配水全局变量.vi" "MB session in"(w232) -> ()
          }
          frame "读状态" {
            # "压力传感器\n4-20  mA \n \n0-8191\n\n0-1MPA"
            n146 = call <vilib>:"Read Holding Registers.vi"("error in (no error)"=w369, "quantity"=u16 80 ("number of holding registers"), "starting address"=u16 0, "MB session in"=w366) -> ("error out"=w364:errorcluster, "Registers"=w331:u16[], "MB session out"=w365:refnum<class "MB_Master.lvclass">)  [unwired: 5 in]
            "Registers" <- w331
            n147 = Array Subset(array=w331, index=48 ("索引")) -> (w337:u16[])  [unwired: 1 in]
            n148 = Index Array(array=w331, index #1=13 ("索引"), index #20=43 ("索引"), index #22=34 ("索引")) -> (element #1=→"R13":u16, element #2=→"R14":u16, element #3=→"R15":u16, element #4=→"R16":u16, element #5=→"R17":u16, element #6=→"R18":u16, element #7=→"R19":u16, element #8=→"R20":u16, element #9=→"R21":u16, element #10=→"R22":u16, element #11=→"R23":u16, element #12=→"R24":u16, element #13=→"R25":u16, element #14=→"R26":u16, element #15=→"R27":u16, element #16=→"R28":u16, element #17=→"R29":u16, element #18=→"R30":u16, element #19=→"R31":u16, element #20=→"R43":u16, element #21=→"R44":u16, element #22=→"R34":u16)  [unwired: 19 in]
            n149 = call <vilib>:"Read Holding Registers.vi"("error in (no error)"=w364, "quantity"=u16 6 ("number of holding registers"), "starting address"=u16 3840, "MB session in"=w365) -> ("error out"=w360:errorcluster, "Registers"=w340:u16[], "MB session out"=w361:refnum<class "MB_Master.lvclass">)  [unwired: 5 in]
            n150 = Array To Cluster(array=w331) -> (cluster=w310:T17)
            n151 = global write "采配水全局变量.vi" "状态"(w310) -> ()
            n152 = To Word Integer(number=w340) -> (16bit integer=w339:i16[])
            n153 = Array To Cluster(array=w340) -> (cluster=w375:T18)
            n154 = global write "采配水全局变量.vi" "AD"(w375) -> ()
            n155 = call <vilib>:"Read Coils.vi"("error in (no error)"=w360, "quantity"=u16 40 ("number of coils"), "starting address"=u16 0, "MB session in"=w361) -> ("error out"=w356:errorcluster, "Coils"=w343:bool[], "MB session out"=w357:refnum<class "MB_Master.lvclass">)  [unwired: 5 in]
            n156 = call "FATEK_HexToString.vi"("数组"=w337) -> ("STRING"=w336:string[])  [unwired: 10 in]
            n157 = global write "采配水全局变量.vi" "输出状态"(w343) -> ()
            n158 = Index Array(array=w336) -> (element=→"采配水版本号":string)  [unwired: 1 in]
            n159 = Index Array(array=w343, index #20=29 ("索引"), index #23=21 ("索引")) -> (element #1=w288:bool, element #2=w287:bool, element #3=w286:bool, element #4=w285:bool, element #5=w284:bool, element #6=w283:bool, element #7=w282:bool, element #8=w281:bool, element #9=w334:bool, element #10=w333:bool, element #11=w280:bool, element #12=w279:bool, element #13=w278:bool, element #14=w277:bool, element #15=w269:bool, element #16=w276:bool, element #17=w275:bool, element #18=w274:bool, element #19=w273:bool, element #20=w272:bool, element #21=w271:bool, element #22=w270:bool, element #23=w292:bool)  [unwired: 21 in]
            n160 = formula code="float AD0,AD1,AD2,AD3,AD4,AD5,AD6;\n\nAD0 = IN[0]*0.0213643-74.9947;\nAD1 = IN[1]*0.0152602-24.9962;\nAD2 = IN[2];\nAD3 = IN[3];\nAD4 = IN[4];\nAD5 = IN[5];"("IN"=w339) -> ("AD0"=w373:dbl, "AD1"=w372:dbl, "AD2"=w332:dbl, "AD3"=w296:dbl, "AD4"=w371:dbl, "AD5"=w370:dbl)
            "配水压力" <- w332
            "供水压力" <- w296
            n161 = call <vilib>:"Read Coils.vi"("error in (no error)"=w356, "quantity"=u16 16 ("number of coils"), "starting address"=u16 1000, "MB session in"=w357) -> ("error out"=w352:errorcluster, "Coils"=w348:bool[], "MB session out"=w353:refnum<class "MB_Master.lvclass">)  [unwired: 5 in]
            n162 = global write "采配水全局变量.vi" "输入状态"(w348) -> ()
            n163 = local write "Y0"(w288) -> ()
            n164 = local write "Y1"(w287) -> ()
            n165 = local write "Y2"(w286) -> ()
            n166 = local write "Y3"(w285) -> ()
            n167 = local write "Y4"(w284) -> ()
            n168 = local write "Y5"(w283) -> ()
            n169 = local write "Y6"(w282) -> ()
            n170 = local write "Y7"(w281) -> ()
            n171 = local write "Y8"(w334) -> ()
            n172 = local write "Y9"(w333) -> ()
            n173 = local write "Y10"(w280) -> ()
            n174 = local write "Y11"(w279) -> ()
            n175 = local write "Y12"(w278) -> ()
            n176 = local write "Y13"(w277) -> ()
            n177 = local write "Y14"(w269) -> ()
            n178 = local write "Y15"(w276) -> ()
            n179 = local write "Y16"(w275) -> ()
            n180 = local write "Y17"(w274) -> ()
            n181 = local write "Y18"(w273) -> ()
            n182 = local write "Y29"(w272) -> ()
            n183 = local write "Y30"(w271) -> ()
            n184 = local write "Y31"(w270) -> ()
            n185 = local write "Y21"(w292) -> ()
            n186 = Index Array(array=w348) -> (element #1=→"X0":bool, element #2=→"X1":bool, element #3=→"X2":bool, element #4=→"X3":bool, element #5=→"X4":bool, element #6=→"X5":bool, element #7=w289:bool, element #8=→"X7":bool, element #9=→"X8":bool, element #10=→"X9":bool, element #11=→"X10":bool, element #12=→"X11":bool, element #13=→"X12":bool, element #14=→"X13":bool)  [unwired: 14 in]
            "X6" <- w289
            n187 = call <vilib>:"Read Coils.vi"("error in (no error)"=w352, "quantity"=u16 16 ("number of coils"), "starting address"=u16 2500, "MB session in"=w353) -> ("error out"=w299:errorcluster, "Coils"=w349:bool[], "MB session out"=w308:refnum<class "MB_Master.lvclass">)  [unwired: 5 in]
            n188 = Bundle(w373, w372, w332, w296, w371, w370) -> (w374:cluster{dbl, dbl, dbl, dbl, dbl, dbl})  [unwired: 1 in]
            n189 = global write "采配水全局变量.vi" "报警簇"(w349) -> ()
            n190 = global write "采配水全局变量.vi" "关门信号"(w289) -> ()
            n191 = global write "采配水全局变量.vi" "转换值"(w374) -> ()
            n192 = call <vilib>:"Read Coils.vi"("error in (no error)"=w299, "quantity"=u16 4, "starting address"=u16 2800, "MB session in"=w308) -> ("error out"=w298:errorcluster, "Coils"=w304:bool[], "MB session out"=w307:refnum<class "MB_Master.lvclass">)  [unwired: 5 in]
            n193 = Index Array(array=w304) -> (element #1=w303:bool, element #2=w300:bool, element #3=w291:bool, element #4=w290:bool)  [unwired: 4 in]
            n194 = global write "采配水全局变量.vi" "看门狗启用"(w303) -> ()
            n195 = local write "三级过滤系统"(w300) -> ()
            n196 = global write "采配水全局变量.vi" "河水净化启用"(w290) -> ()
            n197 = local write "63μm反冲洗阀"(w291) -> ()
          }
          frame "读参数" {
            n198 = call <vilib>:"Read Holding Registers.vi"("error in (no error)"=w408, "quantity"=u16 39 ("number of holding registers"), "starting address"=u16 100, "MB session in"=w409) -> ("error out"=w404:errorcluster, "Registers"=w379:u16[], "MB session out"=w405:refnum<class "MB_Master.lvclass">)  [unwired: 5 in]
            n199 = Array To Cluster(array=w379) -> (cluster=w397:T19)
            n200 = Index Array(array=w379, index #1=37 ("索引")) -> (element #1=→"R137":u16, element #2=→"R138":u16)  [unwired: 1 in]
            n201 = global write "采配水全局变量.vi" "参数设置"(w397) -> ()
            n202 = Unbundle(w397) -> ("Registers[0]"=w396:u16, "Registers[1]"=→"R101":u16, "Registers[2]"=→"R102":u16, "Registers[3]"=→"R103":u16, "Registers[4]"=→"R104":u16, "Registers[5]"=→"R105":u16, "Registers[6]"=→"R106":u16, "Registers[7]"=→"R107":u16, "Registers[8]"=→"R108":u16, "Registers[9]"=→"R109":u16, "Registers[10]"=w383:u16, "Registers[11]"=→"R111":u16, "Registers[12]"=→"R112":u16, "Registers[13]"=w393:u16, "Registers[16]"=→"R116":u16, "Registers[17]"=→"R117":u16, "Registers[20]"=→"R120":u16, "Registers[21]"=→"R121":u16, "Registers[22]"=→"R122":u16, "Registers[24]"=→"R124":u16, "Registers[34]"=w381:u16, "Registers[35]"=→"R135":u16, "Registers[36]"=w380:u16)  [unwired: 14 out]
            n203 = local write "R100"(w396) -> ()
            n204 = local write "R110"(w383) -> ()
            n205 = local write "R113"(w393) -> ()
            n206 = local write "R134"(w381) -> ()
            n207 = local write "R136"(w380) -> ()
          }
          frame "多个写入" {
            n208 = Unbundle By Name(w415) -> ("数据"=w414:variant)
            n209 = Variant To Data(type=T13 {"starting address"=0, "holding register values"=[]}, Variant=w414) -> (data=w412:T13)  [unwired: 1 in, 1 out]
            n210 = Unbundle By Name(w412) -> ("starting address"=w411:u16, "holding register values"=w410:u16[])
            n211 = call <vilib>:"Write Multiple Registers.vi"("error in (no error)"=w418, "values"=w410, "starting address"=w411, "MB session in"=w419) -> ("error out"=w417:errorcluster, "MB session out"=w416:refnum<class "MB_Master.lvclass">)  [unwired: 6 in]
          }
          frame "单个写入" {
            n212 = Unbundle By Name(w425) -> ("数据"=w424:variant)
            n213 = Variant To Data(type=T14 {"starting address"=0, "holding register value"=0}, Variant=w424) -> (data=w422:T14)  [unwired: 1 in, 1 out]
            n214 = Unbundle By Name(w422) -> ("starting address"=w421:u16, "holding register value"=w420:u16)
            n215 = call <vilib>:"Write Single Register.vi"("error in (no error)"=w428, "value"=w420, "address"=w421, "MB session in"=w429) -> ("error out"=w427:errorcluster, "MB session out"=w426:refnum<class "MB_Master.lvclass">)  [unwired: 6 in]
          }
          frame "线圈写入" {
            n216 = Unbundle By Name(w435) -> ("数据"=w434:variant)
            n217 = Variant To Data(type=T15 {"starting address"=0, "coil values"=[]}, Variant=w434) -> (data=w432:T15)  [unwired: 1 in, 1 out]
            n218 = Unbundle By Name(w432) -> ("starting address"=w431:u16, "coil values"=w430:bool[])
            n219 = call <vilib>:"Write Multiple Coils.vi"("error in (no error)"=w438, "values"=w430, "starting address"=w431, "MB session in"=w439) -> ("error out"=w437:errorcluster, "MB session out"=w436:refnum<class "MB_Master.lvclass">)  [unwired: 6 in]
          }
          frame "shutdown" {
            n220 = call <vilib>:"Write Single Register.vi"("error in (no error)"=w443, "value"=u16 0, "address"=u16 4047, "MB session in"=w447) -> ("error out"=w442:errorcluster, "MB session out"=w446:refnum<class "MB_Master.lvclass">)  [unwired: 6 in]
            n221 = call-dynamic "Close Session.vi"("error in (no error)"=w442, "MB session in"=w446) -> ("error out"=w448:errorcluster)  [unwired: 9 in]
            n222 = call <vilib>:"Clear Errors.vi"("error in (no error)"=w448) -> ("error out"=w441:errorcluster)  [unwired: 5 in, 1 out]
            n223 = call "调用WinProladder.vi"("错误输入（无错误）"=w441) -> ("错误输出"=w440:errorcluster)  [unwired: 10 in]
          }
        }
      }
      frame Error {
        n224 = Unbundle By Name(w454) -> ("code"=w456:i32)
        n225 = case shown="-1073807343" w456 {
          tunnel: w455 -> [w458 w462]
          tunnel: w454 -> [w457 w464]
          tunnel: [w457 w463] -> w452
          tunnel: [w458 w462] -> w453
          tunnel: w450 -> [_ w461]
          frame Default {
          }
          frame -1073807343 {
            n226 = Flush Queue(queue=w461) -> (queue out=w460:refnum<queue>)  [unwired: 1 in, 2 out]
            n227 = call-dynamic "Close Session.vi"("error in (no error)"=w464, "MB session in"=w462) -> ("error out"=w463:errorcluster)  [unwired: 9 in]
            n228 = disable-structure shown="禁用" {
              disable-tunnel: w460 -> [w465 _]
              frame Disabled {
                n229 = Enqueue Element At Opposite End(queue=w465, element=cluster{"命令":string, "数据":variant} {"命令"="init", "数据"=variant} ("元素")) -> ()  [unwired: 2 in, 3 out]
              }
              frame Enabled {
              }
            }
            n230 = Wait (ms)(milliseconds to wait=u32 2000 ("等待时间（毫秒）")) -> ()  [unwired: 1 out]
          }
        }
        n231 = call <vilib>:"Clear Errors.vi"("error in (no error)"=w452) -> ("error out"=w451:errorcluster)  [unwired: 5 in, 1 out]
      }
    }
    n232 = Unbundle By Name(w213) -> ("status"=w211:bool)
    "通讯故障" <- w211
    n233 = global write "采配水全局变量.vi" "通讯故障"(w211) -> ()
  }
  n234 = property on="多列列表框" class="MCListbox (严格)"("ItemNames"=string[][] [["待机"], ["初始化"], ["水样润洗"], ["一级水样池进样"], ["二级水样池进样"], ["沉淀"], ["氨氮水样池进样"], ["配水"], ["反冲洗"], ["一级采样池储水"], ["结束"]] ("项名")) -> ()  [unwired: 2 in, 2 out]
  n235 = call-dynamic "Close Session.vi"("error in (no error)"=w8, "MB session in"=w7) -> ()  [unwired: 9 in, 1 out]
